vi "Laser-Main-2018-04-27.vi"() -> ()   [LabVIEW 2013]
doc: "Use this template to build a user interface event handler design pattern. Use this pattern for dialog boxes and other user interfaces. You also can create and execute user-defined events that the VI can handle the same way as user interface events."
uses:
  <vilib>/Instr/_visa.llb/VISA Configure Serial Port (Instr).vi
panel:
  in  "ShutDownSystem":bool
  out "LaserState":bool[](array[boolean])
  in  "SetLaserEnergy":dbl=0.8
  in  "LaserHV":u8=20
  in  "LaserFreq":u8=60
  in  "ComForLaser":refnum<visa-resource-name>="COM3"
  in  "Serial Settings":T1={"baud rate"=9600, "data bits"=8, "parity"=enum."None", "stop bits"=10, "flow control"=0} {"flow control" items=["None"=0, "XON/XOFF"=1, "RTS/CTS"=2, "DTR/DSR"=4]; "stop bits" items=["1.0"=10, "1.5"=15, "2.0"=20]; "data bits" min=5 max=8 step=1; "baud rate" items=["75"=75, "110"=110, "134"=134, "150"=150, "300"=300, "600"=600, "1200"=1200, "1800"=1800, "2400"=2400, "4800"=4800, "7200"=7200, "9600"=9600, "14400"=14400, "19200"=19200, "28800"=28800, "38400"=38400, "56000"=56000, "57600"=57600, "115200"=115200, "128000"=128000, "230400"=230400]}
  in  "Off_Laser":bool
  in  "Start_Laser":bool
  # "连接"
  # "待机"
  # "发射"
  # "内存"
  # "测能"
  # "温警"
  # "静态"
  # "操作"
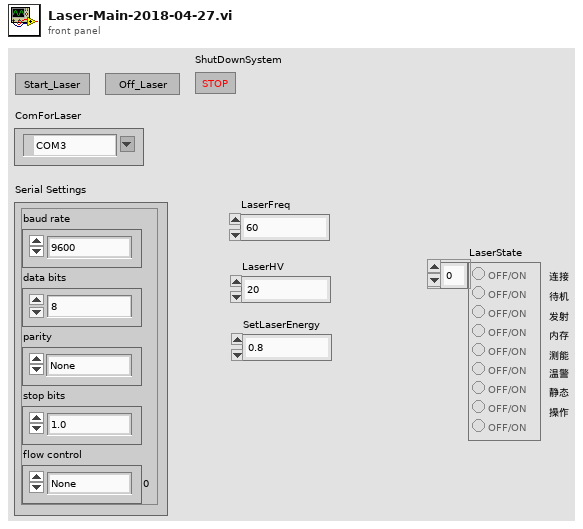
[diagram p1: front panel]
types:
  T1 = cluster{"baud rate":u32, "data bits":u16, "parity":enum16{"None", "Odd", "Even", "Mark", "Space"}, "stop bits":u16, "flow control":u16}
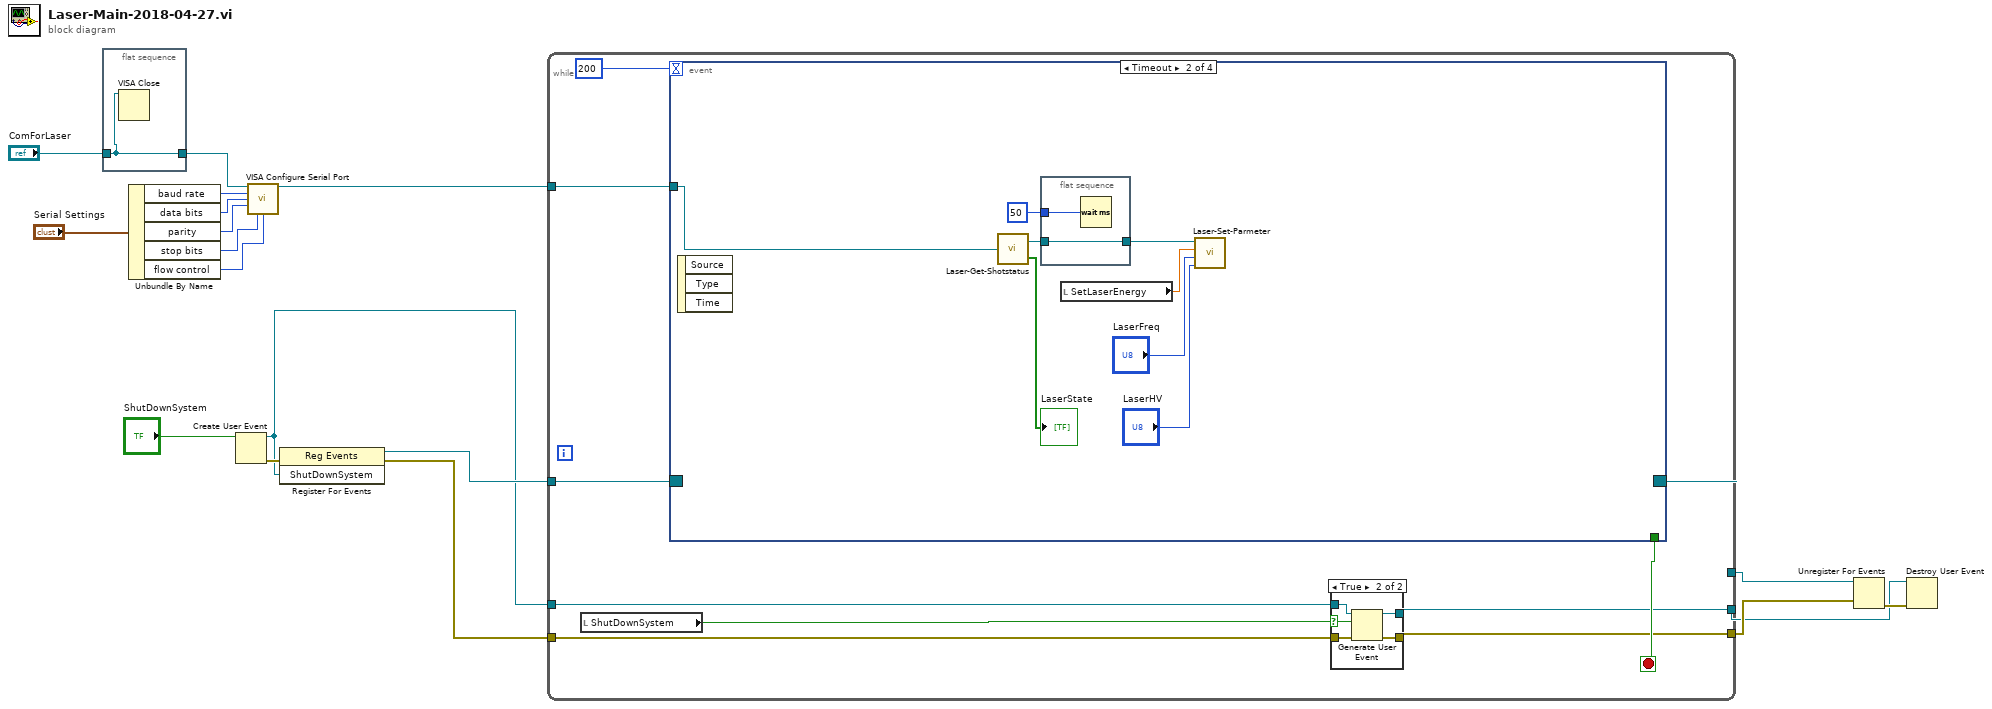
[diagram p0: block diagram]
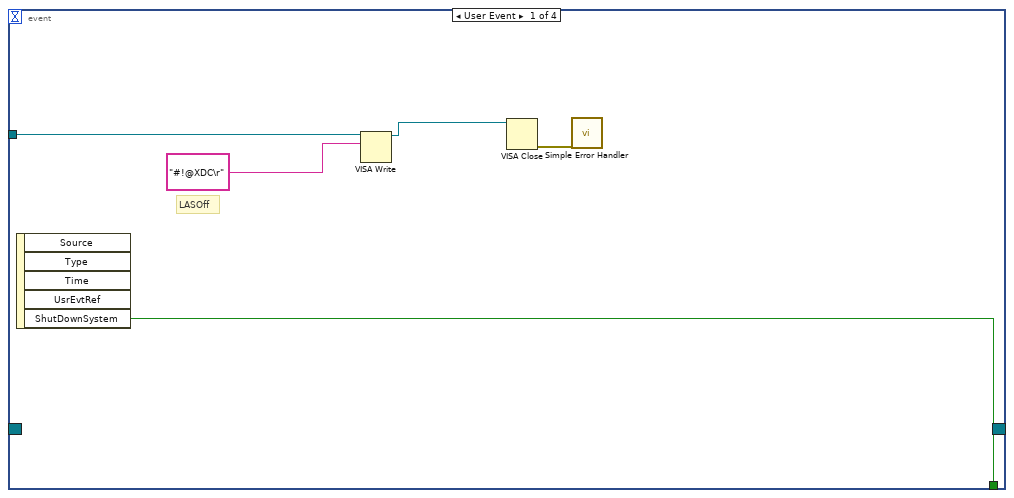
[diagram p3: hidden frame]
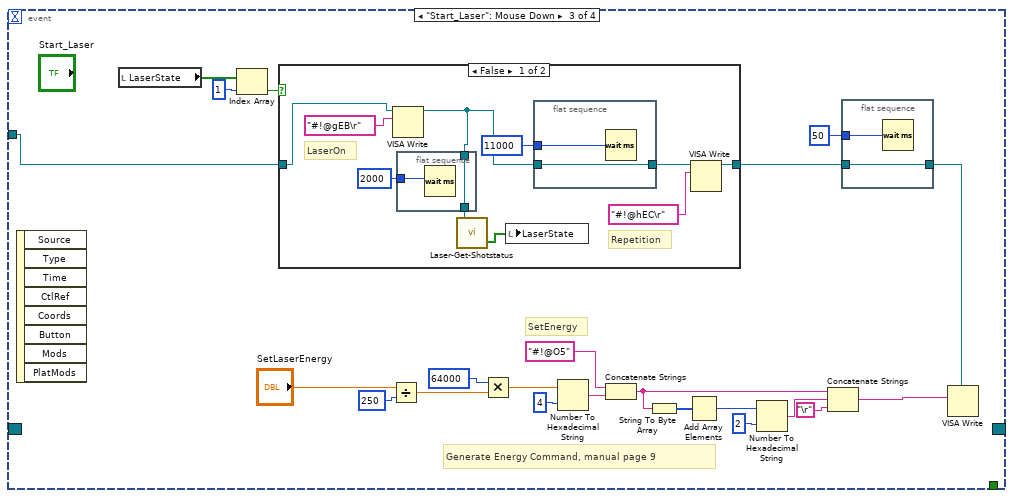
[diagram p4: hidden frame]
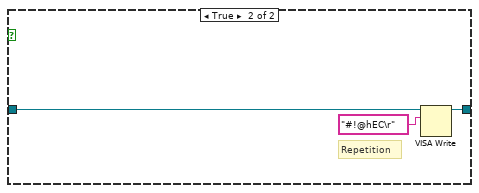
[diagram p5: hidden frame]
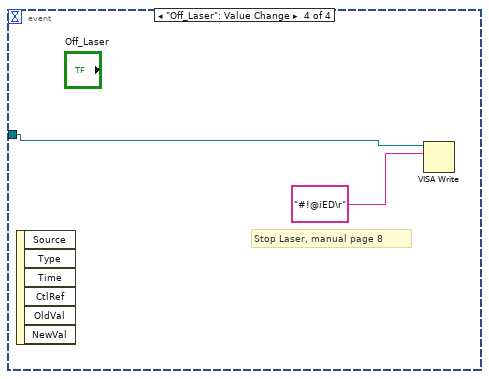
[diagram p6: hidden frame]
diagram:
  n1 = flat-sequence {
    tunnel: "ComForLaser" -> [w19]
    tunnel: [w19] -> w11
    frame #0 {
      n2 = VISA Close(VISA resource name=w19) -> ()  [unwired: 1 in, 1 out]
    }
  }
  n3 = Unbundle By Name("Serial Settings") -> ("baud rate"=w17:u32, "data bits"=w16:u16, "parity"=w15:enum16{"None", "Odd", "Even", "Mark", "Space"}, "stop bits"=w14:u16, "flow control"=w13:u16)
  n4 = Create User Event(user event datatype="ShutDownSystem") -> (user event=w5:refnum<user-event>, error out=w7:errorcluster)  [unwired: 1 in]
  n5 = call-poly "VISA Configure Serial Port"("VISA resource name"=w11, "baud rate (9600)"=w17, "data bits (8)"=w16, "parity (0:none)"=w15, "stop bits (10: 1 bit)"=w14, "flow control (0:none)"=w13) -> ("VISA resource name out"=w10:refnum<visa-resource-name>)  [unwired: 3 in, 6 out]
  n6 = register-events(error in=w7, w5) -> (reference out=w8:refnum<event-registration>, error out=w6:errorcluster)  [unwired: 1 in]
  n7 = while {
    tunnel: w10 -> [w28]
    tunnel: w8 -> [w27]
    tunnel: w6 -> [w25]
    tunnel: w5 -> [w24]
    tunnel: [w22] -> w4
    tunnel: [w21] -> w3
    tunnel: [w20] -> w1
    stop <- w23 stop-if-true
    n8 = local read "ShutDownSystem"() -> (w26:bool)
    n9 = event shown="[1] Timeout" {
      selector: w27 -> [_ _ _ _]
      dyn-events: [_ _ _ _] -> w22
      timeout: 200 -> [_ _ _ _]
      tunnel: w28 -> [w38 w48 w52 w93]
      tunnel: [w37 _ _ _] -> w23
      event User Event {
        # "LASOff"
        n10 = event-data() -> ("ShutDownSystem"=w37:bool)  [unwired: 1 in, 4 out]
        n11 = VISA Write(VISA resource name=w38, write buffer="#!@XDC\r") -> (VISA resource name out=w41:refnum<visa-resource-name>)  [unwired: 1 in, 2 out]
        n12 = VISA Close(VISA resource name=w41) -> (error out=w39:errorcluster)  [unwired: 1 in]
        n13 = call <vilib>:"Simple Error Handler.vi"("error in (no error)"=w39) -> ()  [unwired: 1 in, 8 out]
      }
      event Timeout {
        n14 = event-data() -> ()  [unwired: 1 in, 3 out]
        n15 = call "Laser-Get-Shotstatus.vi"("VISA resource name"=w48) -> ("VISA resource name out"=w46:refnum<visa-resource-name>, "LaserState"=→"LaserState":bool[])
        n16 = flat-sequence {
          tunnel: u32 50 ("delay before read (ms)") -> [w51]
          tunnel: w46 -> [w50]
          tunnel: [w50] -> w45
          frame #0 {
            n17 = Wait (ms)(milliseconds to wait=w51) -> ()  [unwired: 1 out]
          }
        }
        n18 = local read "SetLaserEnergy"() -> (w44:dbl)
        n19 = call "Laser-Set-Parmeter.vi"("LaserHV"="LaserHV", "LaserFreq"="LaserFreq", "SetLaserEnergy"=w44, "VISA resource name"=w45) -> ()  [unwired: 1 out]
      }
      event "Start_Laser": Mouse Down {
        # "Generate Energy Command, manual page 9"
        # "SetEnergy"
        n20 = event-data() -> ()  [unwired: 1 in, 8 out]
        n21 = local read "LaserState"() -> (w73:bool[])
        n22 = Index Array(array=w73, index=1) -> (element=w71:bool)
        n23 = case shown="False" w71 {
          tunnel: w52 -> [w79 w91]
          tunnel: [w81 w90] -> w54
          frame False {
            # "LaserOn"
            # "Repetition"
            n24 = VISA Write(VISA resource name=w79, write buffer="#!@gEB\r") -> (VISA resource name out=w77:refnum<visa-resource-name>)  [unwired: 1 in, 2 out]
            n25 = flat-sequence {
              tunnel: 2000 -> [w87]
              tunnel: w77 -> [w86]
              tunnel: [w86] -> w76
              frame #0 {
                n26 = Wait (ms)(milliseconds to wait=w87) -> ()  [unwired: 1 out]
              }
            }
            n27 = call "Laser-Get-Shotstatus.vi"("VISA resource name"=w76) -> ("LaserState"=w80:bool[])  [unwired: 1 out]
            n28 = local write "LaserState"(w80) -> ()
            n29 = flat-sequence {
              tunnel: w77 -> [w89]
              tunnel: [w89] -> w82
              tunnel: u32 11000 ("delay before read (ms)") -> [w88]
              frame #0 {
                n30 = Wait (ms)(milliseconds to wait=w88) -> ()  [unwired: 1 out]
              }
            }
            n31 = VISA Write(VISA resource name=w82, write buffer="#!@hEC\r") -> (VISA resource name out=w81:refnum<visa-resource-name>)  [unwired: 1 in, 2 out]
          }
          frame True {
            # "Repetition"
            n32 = VISA Write(VISA resource name=w91, write buffer="#!@hEC\r") -> (VISA resource name out=w90:refnum<visa-resource-name>)  [unwired: 1 in, 2 out]
          }
        }
        n33 = Divide(x="SetLaserEnergy", y=250) -> (x/y=w59:dbl)
        n34 = Multiply(x=64000, y=w59) -> (x*y=w57:dbl)
        n35 = Number To Hexadecimal String(1:i16 4 ("width (-)"), 2:w57) -> (0:w68:string)
        n36 = Concatenate Strings("#!@O5" ("string"), w68) -> (w64:string)
        n37 = String To Byte Array(string=w64) -> (unsigned byte array=w67:u8[])
        n38 = Add Array Elements(numeric array=w67) -> (sum=w66:u8)
        n39 = Number To Hexadecimal String(1:i16 2 ("width (-)"), 2:w66) -> (0:w63:string)
        n40 = Concatenate Strings(w64, w63, "\r") -> (w55:string)
        n41 = flat-sequence {
          tunnel: u32 50 ("delay before read (ms)") -> [w75]
          tunnel: w54 -> [w74]
          tunnel: [w74] -> w53
          frame #0 {
            n42 = Wait (ms)(milliseconds to wait=w75) -> ()  [unwired: 1 out]
          }
        }
        n43 = VISA Write(VISA resource name=w53, write buffer=w55) -> ()  [unwired: 1 in, 3 out]
      }
      event "Off_Laser": Value Change {
        # "Stop Laser, manual page 8"
        n44 = event-data() -> ()  [unwired: 1 in, 6 out]
        n45 = VISA Write(VISA resource name=w93, write buffer="#!@iED\r") -> ()  [unwired: 1 in, 3 out]
      }
    }
    n46 = case shown="True" w26 {
      selector: w26 -> [_ w34]
      tunnel: w25 -> [w30 w36]
      tunnel: w24 -> [w31 w35]
      tunnel: [w30 w33] -> w21
      tunnel: [w31 w32] -> w20
      frame False {
      }
      frame True {
        n47 = Generate User Event(user event=w35, event data cluster=w34, error in=w36) -> (user event out=w32:refnum<user-event>, error out=w33:errorcluster)  [unwired: 1 in]
      }
    }
  }
  n48 = Unregister For Events(event registration refnum=w4, error in=w3) -> (error out=w2:errorcluster)
  n49 = Destroy User Event(user event=w1, error in=w2) -> ()  [unwired: 1 out]
